vi "Frontend v3.0.vi"() -> ()   [LabVIEW 2016]
uses:
  Driver/Old driver/4155C Filename.vi
panel:
  in  "Panel Controls 2":T1={"Emergency Stop"=refnum, "CapGraph Max"=1e-05, "Text/Graph (text=false)"=FALSE} {"CapGraph Max" format="%.2e"}
  in  "Gate 3":T2={"Gate Start"=0.0, "Gate Stop"=2.0, "Gate Step"=1.0, "Gate Compliance"=0.0001, "Range mode"=0, "Range"=6} {"Range" max=11 scale=0.0..11.0; "Range mode" items=["Auto", "Limited", "Fixed"]; "Gate Compliance" min=0.0 max=0.1 format="%^.2e"; "Gate Step" min=-100.0 max=100.0 format="%^.4e"; "Gate Stop" min=-100.0 max=100.0 format="%^.4e"; "Gate Start" min=-100.0 max=100.0 format="%^.4e"}
  in  "Drain 3":T3={"Drain voltage"=0.0, "Drain Compliance"=0.0001, "Range mode"=0, "Range"=6} {"Range" max=11 scale=0.0..11.0; "Range mode" items=["Auto", "Limited", "Fixed"]; "Drain Compliance" min=0.0 max=0.1 format="%^.2e"; "Drain voltage" min=-100.0 max=100.0 format="%^.4e"}
  in  "Timings 2":T4={"hold time (sec)"=0.0, "delay time (sec)"=0.0, "Step Time (0 disables)"=0.0, "C-Step"=0.1, "CInt"=0.1, "IInt"=0.1} {"IInt" min=0.01 max=10.0 format="%.2f"; "CInt" min=0.01 max=10.0 format="%.2f"; "C-Step" min=0.01 max=10.0 format="%.2f"; "Step Time (0 disables)" min=0.0 format="%.2f"; "delay time (sec)" min=0.0 format="%.4f"; "hold time (sec)" min=0.0 format="%.4f"}
  in  "Gate 2":T5={"Gate Start"=0.0, "Gate Stop"=2.0, "Gate Step (linear only)"=1.0, "Gate Compliance"=0.0001, "Gate PComp"=0.0, "Range mode"=0, "Range"=6} {"Range" max=11 scale=0.0..11.0; "Range mode" items=["Auto", "Limited", "Fixed"]; "Gate PComp" format="%^.2e"; "Gate Compliance" format="%^.2e"; "Gate Step (linear only)" format="%^.4e"; "Gate Stop" format="%^.4e"; "Gate Start" format="%^.4e"}
  in  "Drain":T6={"Drain Start"=0.0, "Drain Stop"=2.0, "Drain Compliance"=0.0001, "Drain Step"=1.0, "Drain PComp"=0.0, "Range mode"=0, "Range"=6} {"Range" max=11 scale=0.0..11.0; "Range mode" items=["Auto", "Limited", "Fixed"]; "Drain PComp" format="%^.2e"; "Drain Step" format="%^.4e"; "Drain Compliance" format="%^.2e"; "Drain Stop" format="%^.4e"; "Drain Start" format="%^.4e"}
  in  "Gate":T7={"Gate Start"=0.0, "Gate Stop"=2.0, "Gate Step"=1.0, "Gate Compliance"=0.0001, "Gate PComp"=0.0, "Range mode"=0, "Range"=6} {"Range" max=11 scale=0.0..11.0; "Range mode" items=["Auto", "Limited", "Fixed"]; "Gate PComp" format="%^.2e"; "Gate Compliance" format="%^.2e"; "Gate Step" format="%^.4e"; "Gate Stop" format="%^.4e"; "Gate Start" format="%^.4e"}
  in  "Drain 2":T8={"Drain Start"=0.0, "Drain Stop"=2.0, "Drain Compliance"=0.0001, "Drain Step (linear only)"=1.0, "Drain PComp"=0.0, "Range mode"=0, "Range"=6} {"Range" max=11 scale=0.0..11.0; "Range mode" items=["Auto", "Limited", "Fixed"]; "Drain PComp" format="%^.2e"; "Drain Step (linear only)" format="%^.4e"; "Drain Compliance" format="%^.2e"; "Drain Stop" format="%^.4e"; "Drain Start" format="%^.4e"}
  in  "Timings":T9={"integration time"=0, "Short/Long integration time"=0.00064, "hold time (sec)"=0.0, "delay time (sec)"=0.0, "Step Time (0 disables)"=0.0, "sweep method"=0, "Pulse period"=0.005, "Base voltage"=0.0, "Pulse width"=0.0005} {"Pulse width" min=0.0005 max=0.1 step=0.0001 format="%.4f"; "Base voltage" format="%^.4e"; "Pulse period" min=0.005 max=1.0 step=0.0001 format="%.4f"; "sweep method" items=["Continuous", "Pulsed"]; "Step Time (0 disables)" format="%.2f"; "delay time (sec)" format="%.4f"; "hold time (sec)" format="%.4f"; "Short/Long integration time" format="%^.0e"; "integration time" scale=0.0..2.0}
  in  "Panel controls":T10={"Emergency Stop"=refnum, "OutputGraph Max"=1e-05, "Text/Graph (text=false)"=FALSE} {"OutputGraph Max" format="%.2e"}
  in  "Panel Controls":T11={"Emergency Stop"=refnum, "TransGraph Max"=1e-05, "Text/Graph (text=false)"=FALSE, "TransGraph Min"=1e-05} {"TransGraph Min" format="%.2e"; "TransGraph Max" format="%.2e"}
  in  "Tab Control":enum32{"Characteristics", "Other parameters"}(tab)
  in  "Drain Voltage":dbl min=-100.0 max=100.0 format="%.2f"
  in  "Cap voltage":dbl=0.1 min=0.0 max=10.0 format="%.2f"
  in  "Leak I-time":dbl=0.1 min=0.02 max=2.0 step=0.02 format="%.2f"
  in  "Cap I-time":dbl=0.1 min=0.04 max=400.0 step=0.02 format="%.2f"
  in  "QSCV Start":bool
  in  "Gate: Step 2":dbl=-2.0 format="%.2f"
  in  "Gate: Stop 2":dbl=-60.0 min=-100.0 max=100.0 format="%.2f"
  in  "Gate: Start 2":dbl min=-100.0 max=100.0 format="%.2f"
  in  "sweep method":u16(ring) items=["Continuous", "Pulsed"]
  out "Is":dbl format="%.2e"
  out "Id":dbl format="%.2e"
  out "Ig":dbl format="%.2e"
  in  "Vd":dbl(slide) min=-100.0 max=100.0 step=0.1 scale=-100.0..100.0 scale format="%.1f"
  in  "Vg":dbl(slide) min=-100.0 max=100.0 step=0.1 scale=-100.0..100.0 scale format="%.1f"
  in  "Real time sweep":bool
  in  "Interrupt run":bool
  in  "Running":bool=TRUE
  out "Path":path
  in  "integration time":u32(slide)=1 max=2 step=1 scale=0.0..2.0
  in  "sweep mode":u16(ring)=1 items=["Single", "Double"]
  in  "Transfer Start":bool
  in  "Output Start":bool
  in  "Drain: Step":dbl=1.0 min=-100.0 max=100.0 format="%.2f"
  in  "Drain: Stop":dbl=60.0 min=-100.0 max=100.0 format="%.2f"
  in  "Drain:Start":dbl min=-100.0 max=100.0 format="%.2f"
  in  "Gate: Step":dbl=10.0 min=-100.0 max=100.0 format="%.2f"
  in  "Gate: Stop":dbl=60.0 min=-100.0 max=100.0 format="%.2f"
  in  "Gate: Start":dbl min=-100.0 max=100.0 format="%.2f"
  out "XY Graph":cluster{"Y data in":dbl[], "X data in":dbl[]}[](graph)
  in  "Drain: Step":dbl=-55.0 min=-100.0 max=100.0 format="%.3f"
  in  "Drain: Stop":dbl=-60.0 min=-100.0 max=100.0 format="%.3f"
  in  "Drain:Start":dbl=-5.0 min=-100.0 max=100.0 format="%.3f"
  in  "Gate: Step":dbl=-1.0 min=-100.0 max=100.0 format="%.2f"
  in  "Gate: Stop":dbl=-60.0 min=-100.0 max=100.0 format="%.2f"
  in  "Gate: Start":dbl=10.0 min=-100.0 max=100.0 format="%.2f"
  in  "Gate: Compliance":dbl=0.001 min=1e-12 max=0.1 format="%.8f"
  in  "Drain: Compliance":dbl=0.01 min=1e-12 max=0.1 format="%.8f"
  in  "Drain":u32(ring)=1 items=["SMU1  ", "SMU2  ", "SMU3  ", "SMU4  ", "SMU5  ", "SMU6  ", "VSU1  ", "VSU2  "]
  in  "Source/Common":u32(ring) items=["SMU1  ", "SMU2  ", "SMU3  ", "SMU4  ", "SMU5  ", "SMU6  ", "VSU1  ", "VSU2  "]
  in  "Gate":u32(ring)=2 items=["SMU1  ", "SMU2  ", "SMU3  ", "SMU4  ", "SMU5  ", "SMU6  ", "VSU1  ", "VSU2  "]
  in  "Probe 4":u32(ring)=3 items=["SMU1  ", "SMU2  ", "SMU3  ", "SMU4  ", "SMU5  ", "SMU6  ", "VSU1  ", "VSU2  "]
  in  "TransGraph Min":dbl=1e-11 format="%.2e"
  in  "Logfile?":bool
  in  "Probe 4":cluster{"on/off":bool, "Voltage":dbl} {"Voltage" min=-100.0 max=100.0 format="%.2f"}
  in  "Pulse width":dbl=0.02 min=0.0005 max=0.1 step=0.0001 format="%.4f"
  in  "Base voltage":dbl min=-100.0 max=100.0 format="%.2f"
  in  "Pulse period":dbl=0.5 min=0.005 max=1.0 step=0.0001 format="%.4f"
  in  "Source/Drain\nRange":u8(slide)=3 max=11 scale=0.0..11.0
  in  "Source/Drain\nRange mode":u16(ring)=1 items=["Auto", "Limited", "Fixed"]
  in  "Gate Range":u8(slide)=3 max=11 scale=0.0..11.0
  in  "Gate Range\nmode":u16(ring)=1 items=["Auto", "Limited", "Fixed"]
  in  "Drain Power Compliance":dbl min=0.0 max=1.0 format="%.2f"
  in  "Gate Power\nCompliance":dbl min=0.0 max=1.0 format="%.2f"
  in  "OutputGraph Max":dbl=0.0001 format="%.2e"
  in  "TransGraph Max":dbl=0.001 format="%.2e"
  in  "SPA Display":bool=TRUE
  in  "Step delay /s":dbl min=0.0 max=1.0 format="%.2f"
  in  "Integration time (long)":dbl=0.32 min=0.04 max=2.0 step=0.02 format="%.2f"
  in  "Integration time (short)":dbl=0.00096 min=8e-05 max=0.00192 step=8e-05 format="%^.0e"
  in  "hold time /s":dbl min=0.0 max=655.35 step=0.01 format="%.2f"
  in  "delay time /s":dbl min=0.0 max=65.535 step=0.0001 format="%.2f"
  in  "Decimal places in header":i8=1
  out "error out":errorcluster
  in  "VISA resource name in":refnum<visa-resource-name>="GPIB0::14::INSTR"
  in  "Standby":T12
  # "Transfer Characteristics"
  # "V"
  # "V"
  # "V"
  # "Gate"
  # "V"
  # "V"
  # "Drain"
  # "V"
  # "Output Characteristics"
  # "V"
  # "V"
  # "V"
  # "Gate"
  # "V"
  # "V"
  # "Drain"
  # "V"
  # "Quasi Static Capacitance measurement"
  # "V"
  # "V"
  # "V"
  # "Gate"
  # "s"
  # "V"
  # "V"
  # "s"
  # "A"
  # "A"
  # "Pulsed mode settings"
  # "s"
  # "NOTE - THIS OVERRIDES THE COMPLIANCE VALUES!"
  # "s"
  # "A"
  # "Enter max power in Watts (max 1W)"
  # "A"
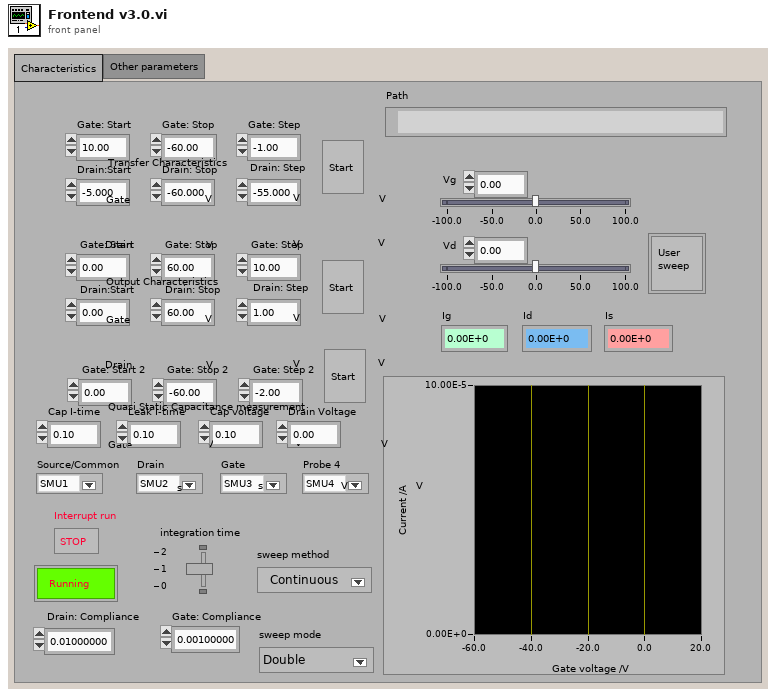
[diagram p1: front panel]
types:
  T1 = cluster{"Emergency Stop":refnum<vi>, "CapGraph Max":dbl, "Text/Graph (text=false)":bool}
  T2 = cluster{"Gate Start":dbl, "Gate Stop":dbl, "Gate Step":dbl, "Gate Compliance":dbl, "Range mode":u16, "Range":u8}
  T3 = cluster{"Drain voltage":dbl, "Drain Compliance":dbl, "Range mode":u16, "Range":u8}
  T4 = cluster{"hold time (sec)":dbl, "delay time (sec)":dbl, "Step Time (0 disables)":dbl, "C-Step":dbl, "CInt":dbl, "IInt":dbl}
  T5 = cluster{"Gate Start":dbl, "Gate Stop":dbl, "Gate Step (linear only)":dbl, "Gate Compliance":dbl, "Gate PComp":dbl, "Range mode":u16, "Range":u8}
  T6 = cluster{"Drain Start":dbl, "Drain Stop":dbl, "Drain Compliance":dbl, "Drain Step":dbl, "Drain PComp":dbl, "Range mode":u16, "Range":u8}
  T7 = cluster{"Gate Start":dbl, "Gate Stop":dbl, "Gate Step":dbl, "Gate Compliance":dbl, "Gate PComp":dbl, "Range mode":u16, "Range":u8}
  T8 = cluster{"Drain Start":dbl, "Drain Stop":dbl, "Drain Compliance":dbl, "Drain Step (linear only)":dbl, "Drain PComp":dbl, "Range mode":u16, "Range":u8}
  T9 = cluster{"integration time":u32, "Short/Long integration time":dbl, "hold time (sec)":dbl, "delay time (sec)":dbl, "Step Time (0 disables)":dbl, "sweep method":u16, "Pulse period":dbl, "Base voltage":dbl, "Pulse width":dbl}
  T10 = cluster{"Emergency Stop":refnum<vi>, "OutputGraph Max":dbl, "Text/Graph (text=false)":bool}
  T11 = cluster{"Emergency Stop":refnum<vi>, "TransGraph Max":dbl, "Text/Graph (text=false)":bool, "TransGraph Min":dbl}
  T12 = cluster{"Gate Standby":bool, "Drain Standby":bool}
  T13 = cluster{"V2 Start":dbl, "V2 Step":dbl, "Number of points":i32}
  T14 = enum16{"open", "replace", "create", "open or create", "replace or create", "replace or create with confirmation"}
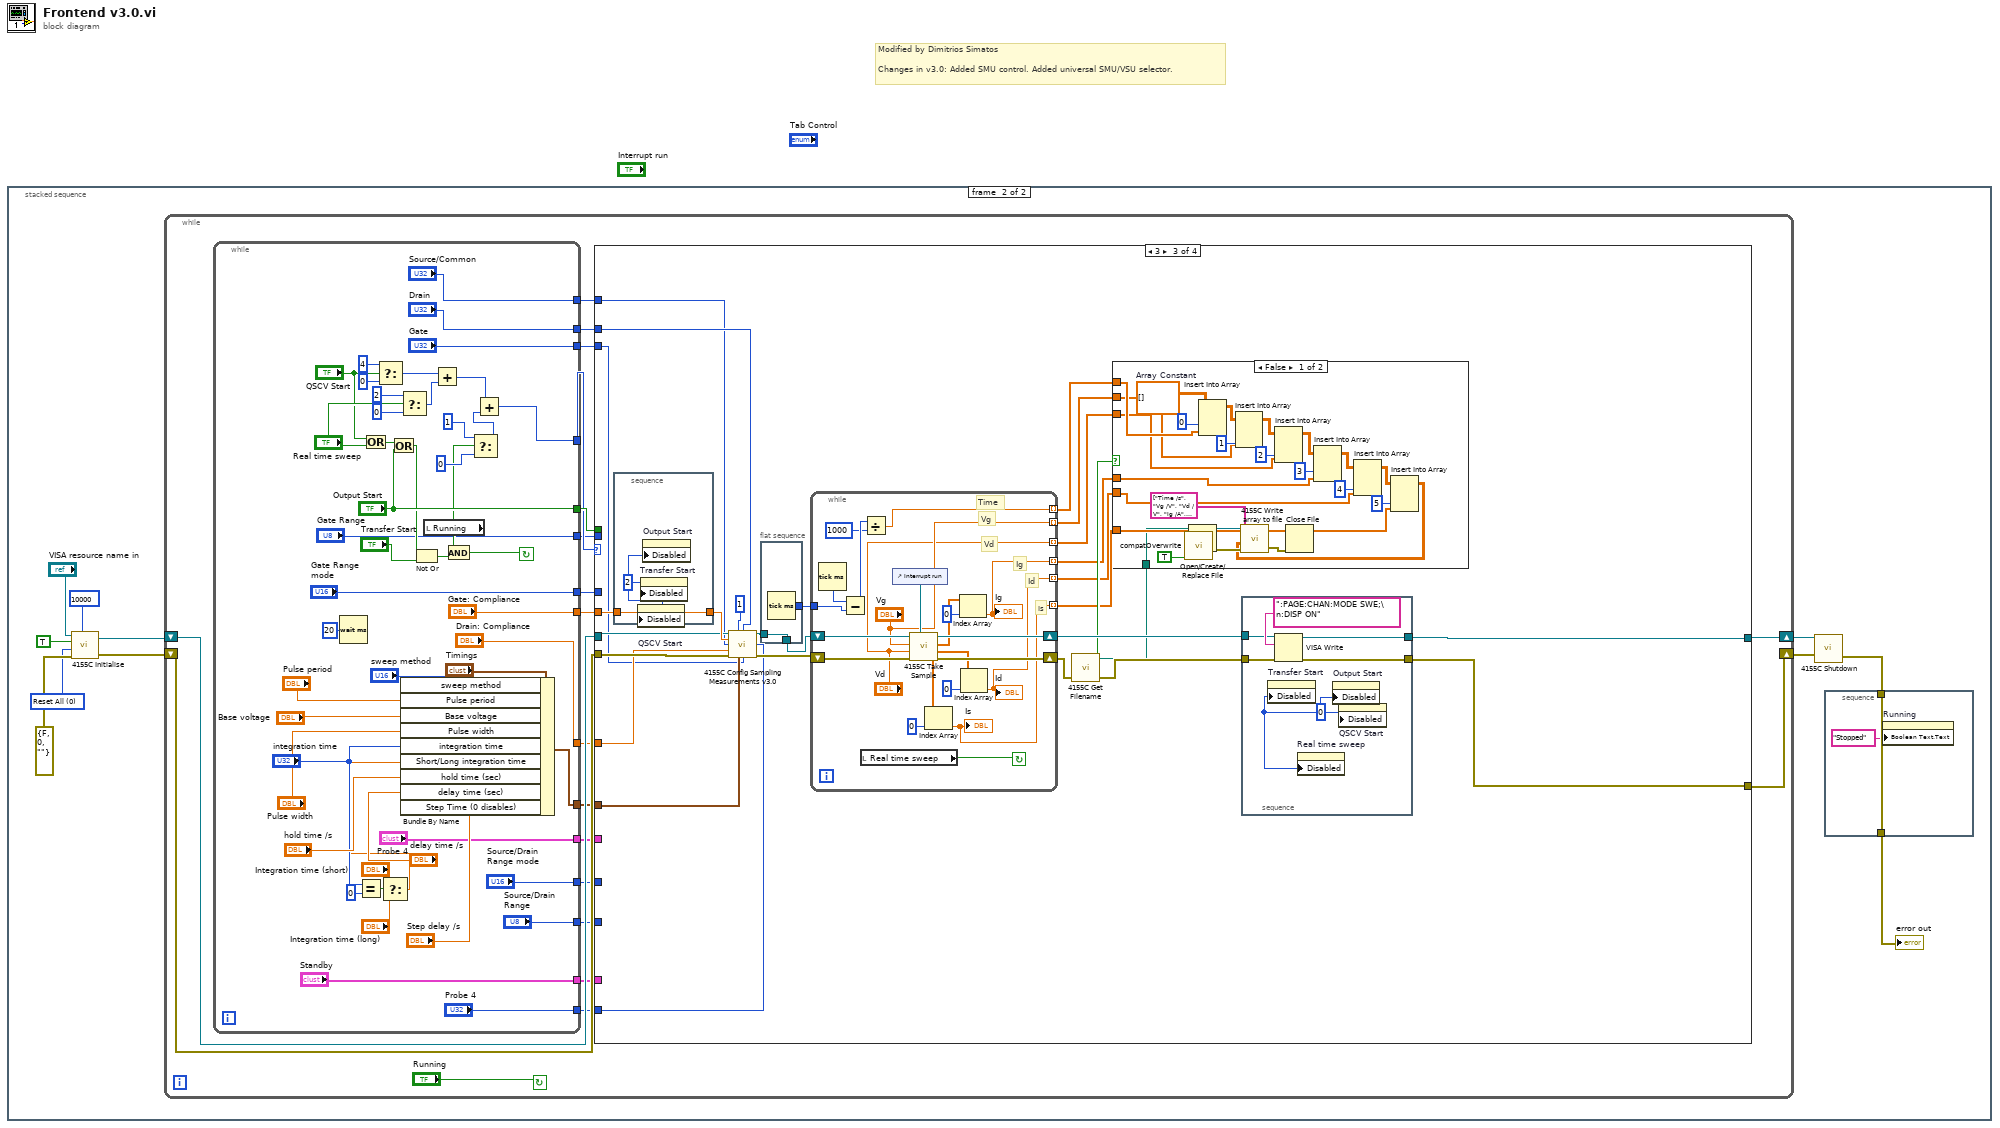
[diagram p0: block diagram]
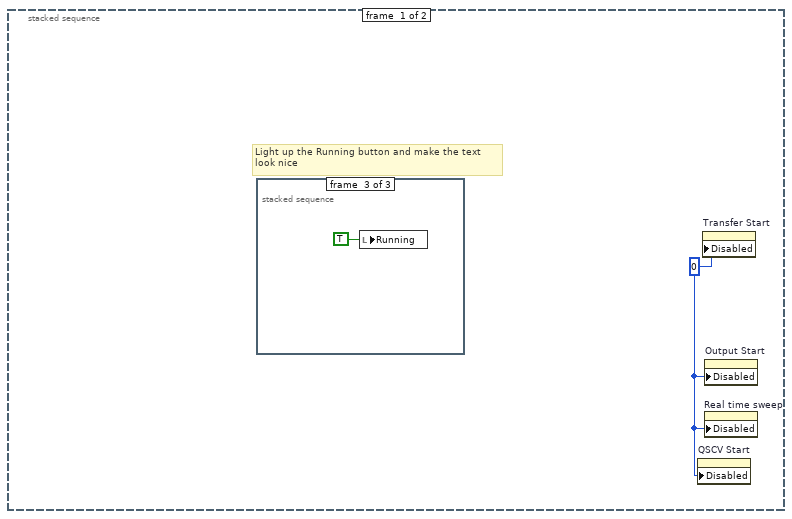
[diagram p2: hidden frame]
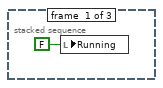
[diagram p3: hidden frame]
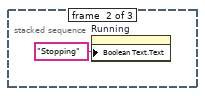
[diagram p4: hidden frame]
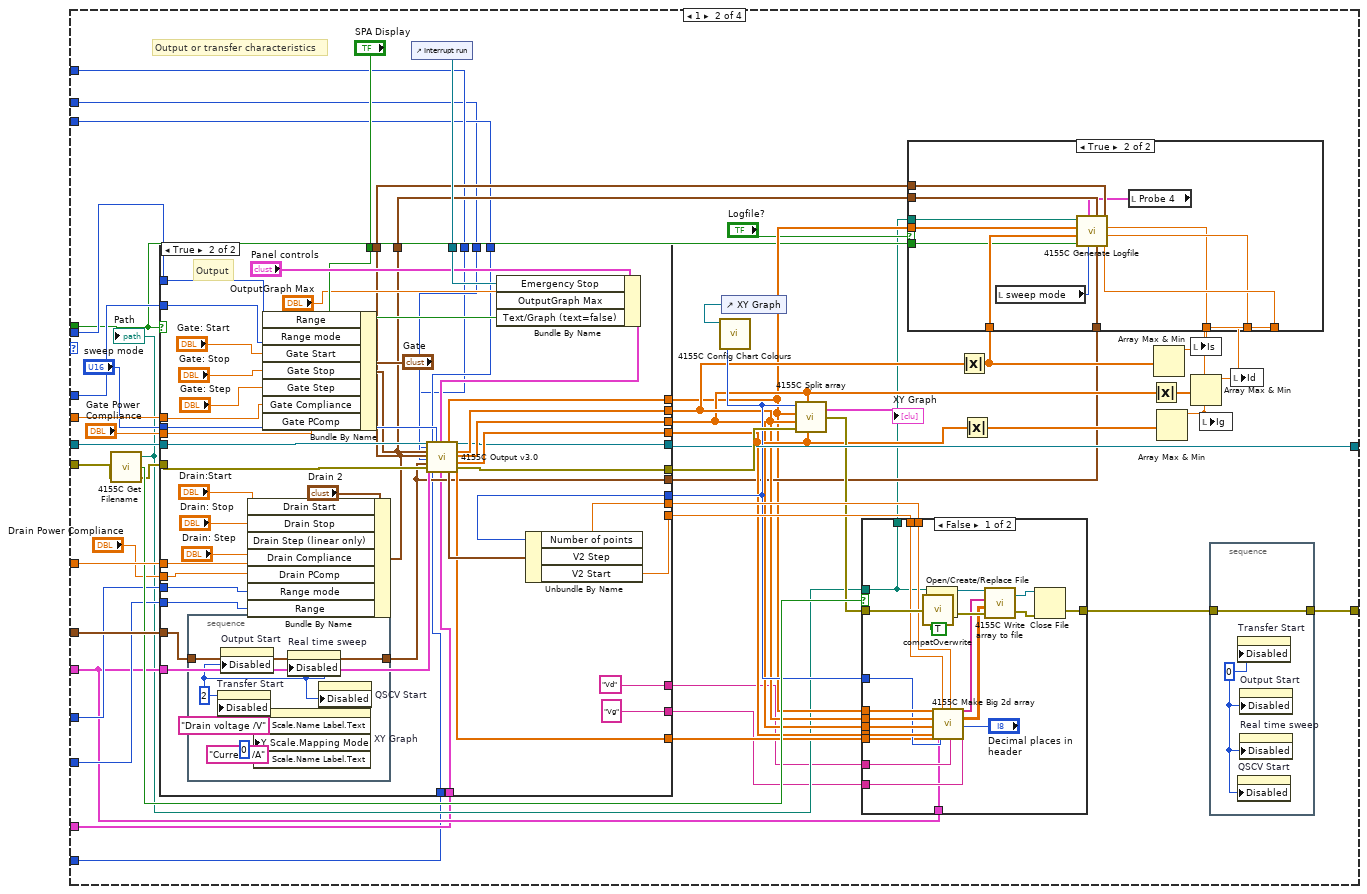
[diagram p6: hidden frame]
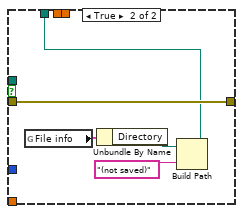
[diagram p8: hidden frame]
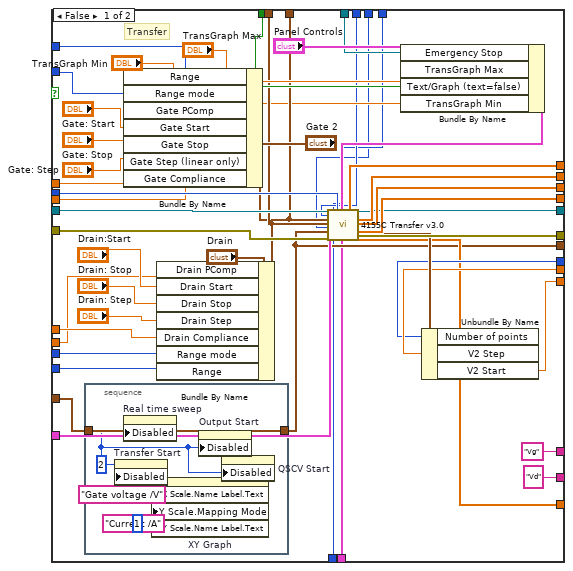
[diagram p9: hidden frame]
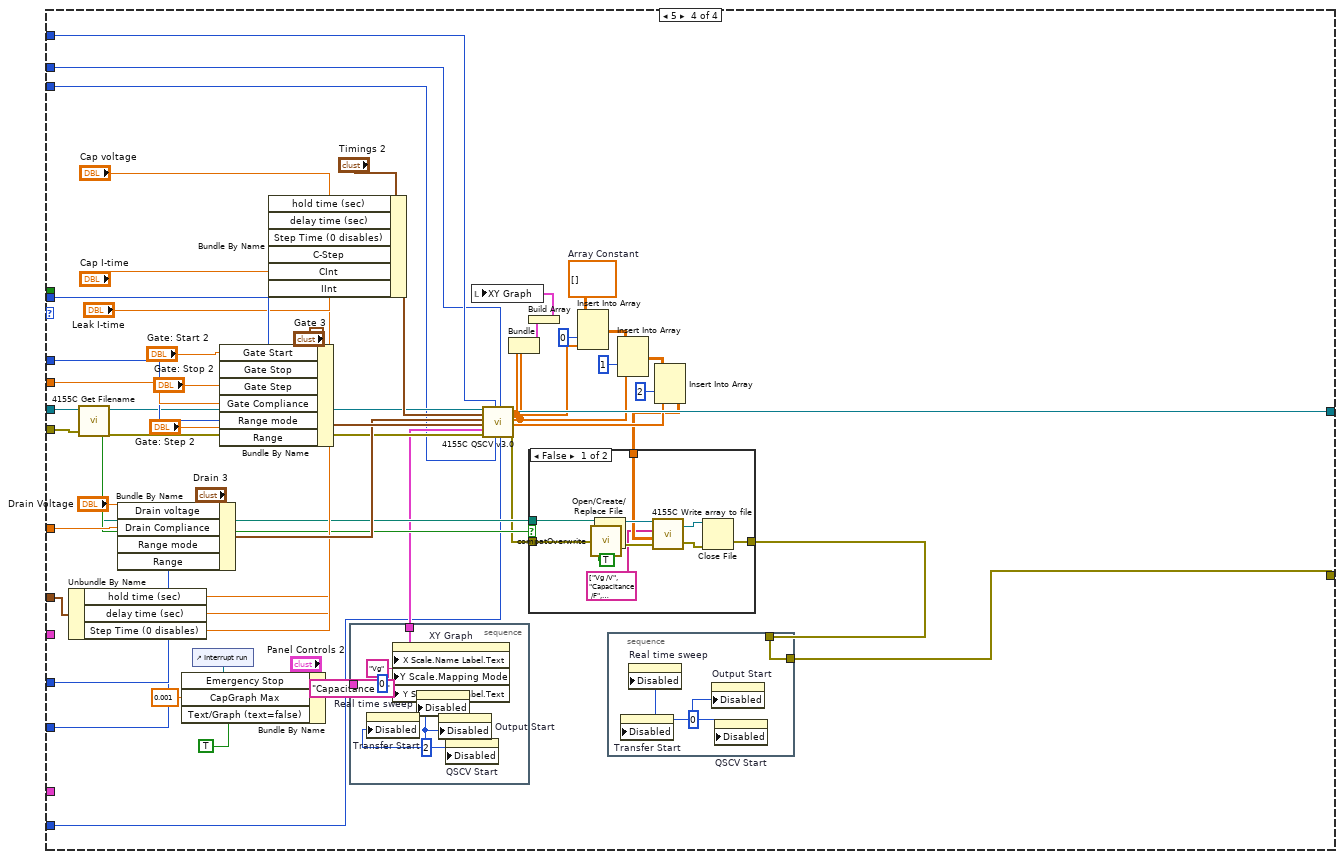
[diagram p11: hidden frame]
diagram:
  # "Modified by Dimitrios Simatos\n\nChanges in v3.0: Added SMU control. Added universal SMU/VSU selector."
  n1 = stacked-sequence {
    frame #0 {
      w1 = u8 0 ("Disabled")
      # "Light up the Running button and make the text\nlook nice"
      n2 = stacked-sequence {
        frame #0 {
          n3 = local write "Running"(FALSE ("Running")) -> ()
        }
        frame #1 {
          n4 = property on="Running" class="Bool (strict)"("Boolean Text.Text"="Stopping") -> ()  [unwired: 2 in, 2 out]
        }
        frame #2 {
          (unwired) FALSE ("Running")
          n5 = local write "Running"(TRUE ("Running")) -> ()
        }
      }
      n6 = property on="QSCV Start" class="Bool (strict)"("Disabled"=w1) -> ()  [unwired: 2 in, 2 out]
      n7 = property on="Transfer Start" class="Bool (strict)"("Disabled"=w1) -> ()  [unwired: 2 in, 2 out]
      n8 = property on="Output Start" class="Bool (strict)"("Disabled"=w1) -> ()  [unwired: 2 in, 2 out]
      n9 = property on="Real time sweep" class="Bool (strict)"("Disabled"=w1) -> ()  [unwired: 2 in, 2 out]
    }
    frame #1 {
      w11 = u16 0 items=["Reset All", "Partial reset"] ("Type of reset")
      n10 = call "4155C Initialise.vi"("VISA resource name in"="VISA resource name in", "Reset"=TRUE, "Type of reset"=w11, "error in (no error)"=errorcluster {"status"=FALSE, "code"=0, "source"=""}, "VISA Timeout Value"=u32 10000) -> ("VISA Resource Name out"=w10:refnum<visa-resource-name>, "error out"=w9:errorcluster)
      n11 = while {
        shift-left: w10 -> [w30]
        shift-right: [w32] -> w5
        shift-left: w9 -> [w31]
        shift-right: [w33] -> w6
        stop <- "Running" continue-if-true
        n12 = while {
          tunnel: ["Probe 4"] -> w21
          tunnel: ["Gate Range"] -> w22
          tunnel: ["Gate Range\nmode"] -> w23
          tunnel: ["Source/Drain\nRange"] -> w24
          tunnel: ["Source/Drain\nRange mode"] -> w25
          tunnel: ["Drain: Compliance"] -> w26
          tunnel: [w41] -> w27
          tunnel: ["Gate: Compliance"] -> w28
          tunnel: [w73] -> w29
          tunnel: ["Output Start"] -> w34
          tunnel: ["Standby"] -> w20
          tunnel: ["Source/Common"] -> w19
          tunnel: ["Gate"] -> w18
          tunnel: ["Drain"] -> w17
          tunnel: ["Probe 4"] -> w16
          stop <- w82 continue-if-true
          n13 = Wait (ms)(milliseconds to wait=u32 20) -> ()  [unwired: 1 out]
          n14 = Equal?(x="integration time", y=u32 0) -> (x = y?=w65:bool)
          n15 = Or(x="QSCV Start", y="Real time sweep") -> (x .or. y?=w53:bool)
          n16 = Select(t=i8 4, s="QSCV Start", f=i8 0) -> (s? t:f=w48:i8)
          n17 = Select(t="Integration time (short)", s=w65, f="Integration time (long)") -> (s? t:f=w62:dbl)
          n18 = Or(x=w53, y="Output Start") -> (x .or. y?=w79:bool)
          n19 = Select(t=i8 2, s="Real time sweep", f=i8 0) -> (s? t:f=w49:i8)
          n20 = Bundle By Name(cluster="Timings", "sweep method"="sweep method", "Pulse period"="Pulse period", "Base voltage"="Base voltage", "Pulse width"="Pulse width", "integration time"="integration time", "Short/Long integration time"=w62, "hold time (sec)"="hold time /s", "delay time (sec)"="delay time /s", "Step Time (0 disables)"="Step delay /s") -> (w41:T9)
          n21 = Not Or(1:"Transfer Start", 2:w79) -> (0:w81:bool)
          n22 = local read "Running"() -> (w76:bool)
          n23 = Add(x=w48, y=w49) -> (x+y=w47:i8)
          n24 = And(x=w76, y=w81) -> (x .and. y?=w82:bool)
          n25 = Select(t=i8 1, s=w76, f=i8 0) -> (s? t:f=w72:i8)
          n26 = Add(x=w47, y=w72) -> (x+y=w73:i8)
        }
        n27 = case shown="3" w29 {
          tunnel: w34 -> [_ w96 _ _]
          tunnel: w27 -> [_ w137 w302 w405]
          tunnel: w28 -> [_ w136 w312 w417]
          tunnel: w26 -> [_ w135 w306 w421]
          tunnel: [w85 w128 w310 w376] -> w33
          tunnel: [w84 w131 w311 w401] -> w32
          tunnel: w31 -> [w85 w122 w308 w397]
          tunnel: w30 -> [w84 w130 w307 w396]
          tunnel: w25 -> [_ w107 _ w414]
          tunnel: w24 -> [_ w106 _ w413]
          tunnel: w23 -> [_ w105 _ w416]
          tunnel: w22 -> [_ w104 _ w415]
          tunnel: w21 -> [_ w102 _ _]
          tunnel: w20 -> [_ w90 _ _]
          tunnel: w19 -> [_ w89 w287 w373]
          tunnel: w18 -> [_ w88 w286 w374]
          tunnel: w17 -> [_ w87 w288 w372]
          tunnel: w16 -> [_ w86 w285 w375]
          frame 0, Default {
            # "Someone's deselected the running button so just shutdown..."
          }
          frame 1 {
            # "Output or transfer characteristics"
            n28 = call "4155C Get Filename.vi"("error in (no error)"=w122) -> ("error out"=w121:errorcluster, "cancelled"=w127:bool, "path"=w95:path)  [unwired: 2 in]
            "Path" <- w95
            n29 = control-ref of="Interrupt run"() -> (w123:refnum<vi>)
            n30 = case shown="True" w96 {
              tunnel: w130 -> [w209 w261]
              tunnel: w121 -> [w208 w260]
              tunnel: w137 -> [w212 w266]
              tunnel: w136 -> [w222 w277]
              tunnel: w135 -> [w227 w276]
              tunnel: "sweep mode" -> [w221 w275]
              tunnel: [w220 w274] -> w97
              tunnel: [w219 w273] -> w109
              tunnel: [w218 w272] -> w108
              tunnel: [w217 w271] -> w110
              tunnel: [w216 w270] -> w131
              tunnel: [w215 w269] -> w134
              tunnel: [w192 w245] -> w126
              tunnel: [w193 w244] -> w132
              tunnel: [w185 w243] -> w133
              tunnel: ["Vg" "Vd"] -> w92
              tunnel: ["Vd" "Vg"] -> w91
              tunnel: w123 -> [w206 w259]
              tunnel: "SPA Display" -> [w205 w257]
              tunnel: "Drain Power Compliance" -> [w201 w254]
              tunnel: "Gate Power\nCompliance" -> [w202 w253]
              tunnel: w107 -> [w196 w250]
              tunnel: w106 -> [w195 w249]
              tunnel: w105 -> [w197 w248]
              tunnel: w104 -> [w198 w247]
              tunnel: w102 -> [w191 w242]
              tunnel: [w190 w241] -> w103
              tunnel: [w189 w239] -> w100
              tunnel: [w188 w240] -> w99
              tunnel: [w187 w238] -> w98
              tunnel: w90 -> [w184 w233]
              tunnel: w89 -> [w183 w235]
              tunnel: w88 -> [w182 w237]
              tunnel: w87 -> [w181 w236]
              tunnel: w86 -> [w180 w234]
              frame False {
                # "Transfer"
                n31 = stacked-sequence {
                  tunnel: w212 -> [w231]
                  tunnel: [w231] -> w187
                  frame #0 {
                    w229 = u8 2 ("Disabled")
                    n32 = property on="Transfer Start" class="Bool (strict)"("Disabled"=w229) -> ()  [unwired: 2 in, 2 out]
                    n33 = property on="Real time sweep" class="Bool (strict)"("Disabled"=w229) -> ()  [unwired: 2 in, 2 out]
                    n34 = property on="XY Graph" class="XYGraph (strict)"("X Scale.Name Label.Text"="Gate voltage /V", "Y Scale.Mapping Mode"=u8 1, "Y Scale.Name Label.Text"="Current /A") -> ()  [unwired: 2 in, 2 out]
                    n35 = property on="Output Start" class="Bool (strict)"("Disabled"=w229) -> ()  [unwired: 2 in, 2 out]
                    n36 = property on="QSCV Start" class="Bool (strict)"("Disabled"=w229) -> ()  [unwired: 2 in, 2 out]
                  }
                }
                n37 = Bundle By Name(cluster="Gate 2", "Range"=w198, "Range mode"=w197, "Gate PComp"=w202, "Gate Start"="Gate: Start", "Gate Stop"="Gate: Stop", "Gate Step (linear only)"="Gate: Step", "Gate Compliance"=w222) -> (w188:T5)
                n38 = Bundle By Name(cluster="Drain", "Drain PComp"=w201, "Drain Start"="Drain:Start", "Drain Stop"="Drain: Stop", "Drain Step"="Drain: Step", "Drain Compliance"=w227, "Range mode"=w196, "Range"=w195) -> (w189:T6)
                n39 = Bundle By Name(cluster="Panel Controls", "Emergency Stop"=w206, "TransGraph Max"="TransGraph Max", "Text/Graph (text=false)"=w205, "TransGraph Min"="TransGraph Min") -> (w203:T11)
                n40 = call "4155C Transfer v3.0.vi"("VISA resource name in"=w209, "Source/Common"=w183, 2:"Gate"=w188, 3:"Drain"=w189, 4:"Drain"=w181, "Timings"=w187, "error in (no error)"=w208, 7:"Probe 4"=w191, 8:"Gate"=w182, 9:"Probe 4"=w180, "sweep mode"=w221, "Panel Controls"=w203, "Standby"=w184) -> ("VG"=w220:dbl[], "Outparams"=w194:T13, "VISA Resource Name out"=w216:refnum<visa-resource-name>, "IS"=w219:dbl[], "ID"=w218:dbl[], "IG"=w217:dbl[], "error out"=w215:errorcluster, "Probe 4"=w190:dbl[])  [unwired: 7 in]
                n41 = Unbundle By Name(w194) -> ("Number of points"=w192:i32, "V2 Step"=w193:dbl, "V2 Start"=w185:dbl)
              }
              frame True {
                # "Output"
                n42 = stacked-sequence {
                  tunnel: w266 -> [w283]
                  tunnel: [w283] -> w238
                  frame #0 {
                    w281 = u8 2 ("Disabled")
                    n43 = property on="Transfer Start" class="Bool (strict)"("Disabled"=w281) -> ()  [unwired: 2 in, 2 out]
                    n44 = property on="Output Start" class="Bool (strict)"("Disabled"=w281) -> ()  [unwired: 2 in, 2 out]
                    n45 = property on="XY Graph" class="XYGraph (strict)"("X Scale.Name Label.Text"="Drain voltage /V", "Y Scale.Mapping Mode"=u8 0, "Y Scale.Name Label.Text"="Current /A") -> ()  [unwired: 2 in, 2 out]
                    n46 = property on="Real time sweep" class="Bool (strict)"("Disabled"=w281) -> ()  [unwired: 2 in, 2 out]
                    n47 = property on="QSCV Start" class="Bool (strict)"("Disabled"=w281) -> ()  [unwired: 2 in, 2 out]
                  }
                }
                n48 = Bundle By Name(cluster="Drain 2", "Drain Start"="Drain:Start", "Drain Stop"="Drain: Stop", "Drain Step (linear only)"="Drain: Step", "Drain Compliance"=w276, "Drain PComp"=w254, "Range mode"=w250, "Range"=w249) -> (w239:T8)
                n49 = Bundle By Name(cluster="Gate", "Range"=w247, "Range mode"=w248, "Gate Start"="Gate: Start", "Gate Stop"="Gate: Stop", "Gate Step"="Gate: Step", "Gate Compliance"=w277, "Gate PComp"=w253) -> (w240:T7)
                n50 = Bundle By Name(cluster="Panel controls", "Emergency Stop"=w259, "OutputGraph Max"="OutputGraph Max", "Text/Graph (text=false)"=w257) -> (w255:T10)
                n51 = call "4155C Output v3.0.vi"("VISA resource name in"=w261, "Source/Common"=w235, 2:"Gate"=w240, 3:"Drain"=w239, 4:"Drain"=w236, "Timings"=w238, "error in (no error)"=w260, 7:"Probe 4"=w242, 8:"Gate"=w237, 9:"Probe 4"=w234, "sweep mode"=w275, "Panel controls"=w255, "Standby"=w233) -> ("VD"=w274:dbl[], "Outparams"=w246:T13, "VISA Resource Name out"=w270:refnum<visa-resource-name>, "IS"=w273:dbl[], "ID"=w272:dbl[], "IG"=w271:dbl[], "error out"=w269:errorcluster, "Probe 4"=w241:dbl[])  [unwired: 7 in]
                n52 = Unbundle By Name(w246) -> ("Number of points"=w245:i32, "V2 Step"=w244:dbl, "V2 Start"=w243:dbl)
              }
            }
            n53 = control-ref of="XY Graph"() -> (w124:refnum<vi>)
            n54 = call "4155C Config Chart Colours.vi"("Numeric"=w126, "XY Graph 2"=w124) -> ()  [unwired: 6 in]
            n55 = call "4155C Split array.vi"("Number of VAR2 steps"=w126, "Y2 data in"=w108, "X data in"=w97, "Y1 data in"=w109, "Y3 data in"=w110, "error in (no error)"=w134) -> ("Array of clusters"=→"XY Graph":cluster{"Y data in":dbl[], "X data in":dbl[]}[], "error out"=w120:errorcluster)  [unwired: 1 in]
            n56 = case shown="False" w127 {
              tunnel: w120 -> [w173 w179]
              tunnel: [w169 w179] -> w129
              tunnel: w95 -> [w153 _]
              tunnel: w126 -> [w163 _]
              tunnel: w108 -> [w165 _]
              tunnel: w97 -> [w167 _]
              tunnel: w109 -> [w166 _]
              tunnel: w110 -> [w164 _]
              tunnel: w133 -> [w157 _]
              tunnel: w132 -> [w158 _]
              tunnel: w92 -> [w162 _]
              tunnel: w91 -> [w161 _]
              tunnel: w103 -> [w155 _]
              tunnel: w102 -> [w154 _]
              tunnel: [w153 w175] -> w93
              frame False {
                n57 = call <vilib>:"compatOverwrite.vi"("overwrite (F)"=TRUE) -> ("overwrite?"=w152:T14)
                n58 = Open/Create/Replace File(file path (use dialog)=w153, error in=w173, operation (0:open)=w152) -> (refnum out=w171:refnum<file>, error out=w172:errorcluster)  [unwired: 3 in, 1 out]
                n59 = call "4155C Make Big 2d array.vi"("1D Var1"=w167, "1d IS"=w166, "1d ID"=w165, "1d IG"=w164, "1d SMU4"=w155, "SMU4"=w154, "VAR2 START"=w157, "Number of VAR2 steps"=w163, "VAR2 STEP"=w158, "VAR1 Name"=w162, "Decimal places in header"="Decimal places in header", "VAR2 Name"=w161) -> ("Header array"=w159:string[], "Data array"=w160:dbl[][])  [unwired: 14 in]
                n60 = call "4155C Write array to file.vi"("Byte Stream File Refnum"=w171, "Header"=w159, "Data Array"=w160, "error in (no error)"=w172) -> ("dup refnum"=w168:refnum<file>, "error out"=w170:errorcluster)  [unwired: 1 in]
                n61 = Close File(refnum=w168, error in=w170) -> (error out=w169:errorcluster)  [unwired: 1 out]
              }
              frame True {
                n62 = global read "4155C Filename.vi" "File info"() -> (w178:cluster{"Filename":string, "Directory":path})
                n63 = Unbundle By Name(w178) -> ("Directory"=w177:path)
                n64 = Build Path(base path=w177, name or relative path="(not saved)") -> (appended path=w175:path)
              }
            }
            n65 = Absolute Value(x=w109) -> (abs(x)=w101:dbl[])
            n66 = Absolute Value(x=w110) -> (abs(x)=w115:dbl[])
            n67 = Absolute Value(x=w108) -> (abs(x)=w114:dbl[])
            n68 = Array Max & Min(array=w101) -> (max value=w112:dbl)  [unwired: 3 out]
            n69 = Array Max & Min(array=w115) -> (max value=w113:dbl)  [unwired: 3 out]
            n70 = local write "Is"(w112) -> ()
            n71 = Array Max & Min(array=w114) -> (max value=w111:dbl)  [unwired: 3 out]
            n72 = case shown="True" "Logfile?" {
              tunnel: w101 -> [_ w146]
              tunnel: w112 -> [_ w142]
              tunnel: w111 -> [_ w143]
              tunnel: w113 -> [_ w144]
              tunnel: w100 -> [_ w149]
              tunnel: w99 -> [_ w148]
              tunnel: w98 -> [_ w147]
              tunnel: w97 -> [_ w145]
              tunnel: w93 -> [_ w139]
              tunnel: w96 -> [_ w138]
              frame False {
              }
              frame True {
                n73 = local read "sweep mode"() -> (w140:u16)
                n74 = local read "Probe 4"() -> (w141:cluster{"on/off":bool, "Voltage":dbl})
                n75 = call "4155C Generate Logfile.vi"("Ig"=w144, "Id"=w143, "Is"=w142, "Drain"=w149, "Timings"=w147, "Gate"=w148, "sweep mode"=w140, "SMU4"=w141, "Output?"=w138, "Input I"=w146, "VG"=w145, "Path"=w139) -> ()
              }
            }
            n76 = local write "Ig"(w113) -> ()
            n77 = stacked-sequence {
              tunnel: w129 -> [w151]
              tunnel: [w151] -> w128
              frame #0 {
                w150 = u8 0 ("Disabled")
                n78 = property on="Transfer Start" class="Bool (strict)"("Disabled"=w150) -> ()  [unwired: 2 in, 2 out]
                n79 = property on="QSCV Start" class="Bool (strict)"("Disabled"=w150) -> ()  [unwired: 2 in, 2 out]
                n80 = property on="Output Start" class="Bool (strict)"("Disabled"=w150) -> ()  [unwired: 2 in, 2 out]
                n81 = property on="Real time sweep" class="Bool (strict)"("Disabled"=w150) -> ()  [unwired: 2 in, 2 out]
              }
            }
            n82 = local write "Id"(w111) -> ()
          }
          frame 3 {
            n83 = stacked-sequence {
              tunnel: w312 -> [w371]
              tunnel: [w371] -> w309
              frame #0 {
                w370 = u8 2 ("Disabled")
                n84 = property on="QSCV Start" class="Bool (strict)"("Disabled"=w370) -> ()  [unwired: 2 in, 2 out]
                n85 = property on="Transfer Start" class="Bool (strict)"("Disabled"=w370) -> ()  [unwired: 2 in, 2 out]
                n86 = property on="Output Start" class="Bool (strict)"("Disabled"=w370) -> ()  [unwired: 2 in, 2 out]
              }
            }
            n87 = call "4155C Config Sampling Measurements v3.0.vi"("VISA session"=w307, "Num Points"=i16 1, "Sample - Drain"=w288, "Gate Compliance"=w309, "Sample - Source/Common"=w287, "Sample - Probe 4"=w285, "Drain Compliance"=w306, "error in (no error)"=w308, "Timings"=w302, "Sample - Gate"=w286) -> ("dup VISA resource name"=w300:refnum<visa-resource-name>, "error out"=w304:errorcluster)  [unwired: 4 in]
            n88 = flat-sequence {
              tunnel: [w341] -> w301
              tunnel: w300 -> [w341]
              tunnel: [w340] -> w299
              frame #0 {
                n89 = Tick Count (ms)() -> (millisecond timer value=w340:u32)
              }
            }
            n90 = while {
              shift-left: w304 -> [w361]
              shift-right: [w360] -> w298
              shift-left: w301 -> [w362]
              shift-right: [w359] -> w305
              tunnel: ["Vg"] -> w293 mode=indexing
              tunnel: ["Vd"] -> w292 mode=indexing
              tunnel: [w349] -> w291 mode=indexing
              tunnel: [w348] -> w290 mode=indexing
              tunnel: [w347] -> w289 mode=indexing
              tunnel: w299 -> [w345]
              tunnel: [w342] -> w294 mode=indexing
              stop <- w363 continue-if-true
              # "Is"
              # "Id"
              # "Ig"
              # "Vd"
              # "Vg"
              # "Time"
              n91 = Tick Count (ms)() -> (millisecond timer value=w346:u32)
              n92 = Subtract(x=w346, y=w345) -> (x-y=w344:u32)
              n93 = local read "Real time sweep"() -> (w363:bool)
              n94 = Divide(x=w344, y=u32 1000) -> (x/y=w342:dbl)
              n95 = control-ref of="Interrupt run"() -> (w358:refnum<vi>)
              n96 = call "4155C Take Sample.vi"("Emergency Stop"=w358, "error in (no error)"=w361, "Vd"="Vd", "Vg"="Vg", "VISA resource name in"=w362) -> ("error out"=w360:errorcluster, "Id"=w354:dbl[], "Ig"=w352:dbl[], "VISA Resource Name out"=w359:refnum<visa-resource-name>, "Is"=w356:dbl[])  [unwired: 1 in, 1 out]
              n97 = Index Array(array=w356, index=0 ("Index")) -> (element=w347:dbl)
              "Is" <- w347
              n98 = Index Array(array=w352, index=0 ("Index")) -> (element=w349:dbl)
              "Ig" <- w349
              n99 = Index Array(array=w354, index=0 ("Index")) -> (element=w348:dbl)
              "Id" <- w348
            }
            n100 = call "4155C Get Filename.vi"("error in (no error)"=w298) -> ("error out"=w297:errorcluster, "cancelled"=w296:bool, "path"=w295:path)  [unwired: 2 in]
            n101 = case shown="False" w296 {
              tunnel: w295 -> [w320 _]
              tunnel: w294 -> [w337 _]
              tunnel: w293 -> [w328 _]
              tunnel: w292 -> [w327 _]
              tunnel: w291 -> [w326 _]
              tunnel: w290 -> [w325 _]
              tunnel: w289 -> [w322 _]
              frame False {
                w339 = dbl[][] []  # Array Constant
                n102 = call <vilib>:"compatOverwrite.vi"("overwrite (F)"=TRUE) -> ("overwrite?"=w313:T14)
                n103 = Open/Create/Replace File(file path (use dialog)=w320, operation (0:open)=w313) -> (refnum out=w318:refnum<file>, error out=w319:errorcluster)  [unwired: 4 in, 1 out]
                n104 = Insert Into Array(array=w339, index (col)=0 ("Disabled Index (col)"), new element=w337) -> (w336:dbl[][])  [unwired: 1 in]
                n105 = Insert Into Array(array=w336, index (col)=1 ("disabled index (col)"), new element=w328) -> (w335:dbl[][])  [unwired: 1 in]
                n106 = Insert Into Array(array=w335, index (col)=2 ("disabled index (col)"), new element=w327) -> (w334:dbl[][])  [unwired: 1 in]
                n107 = Insert Into Array(array=w334, index (col)=3 ("disabled index (col)"), new element=w326) -> (w333:dbl[][])  [unwired: 1 in]
                n108 = Insert Into Array(array=w333, index (col)=4 ("disabled index (col)"), new element=w325) -> (w324:dbl[][])  [unwired: 1 in]
                n109 = Insert Into Array(array=w324, index (col)=5 ("disabled index (col)"), new element=w322) -> (w316:dbl[][])  [unwired: 1 in]
                n110 = call "4155C Write array to file.vi"("Byte Stream File Refnum"=w318, "Header"=string[] ["Time /s", "Vg /V", "Vd /V", "Ig /A", "Id /A", "Is /A"], "Data Array"=w316, "error in (no error)"=w319) -> ("dup refnum"=w317:refnum<file>, "error out"=w321:errorcluster)  [unwired: 1 in]
                n111 = Close File(refnum=w317, error in=w321) -> ()  [unwired: 2 out]
              }
              frame True {
              }
            }
            n112 = stacked-sequence {
              tunnel: [w366] -> w311
              tunnel: [w365] -> w310
              tunnel: w305 -> [w368]
              tunnel: w297 -> [w367]
              frame #0 {
                w364 = u8 0 ("Disabled")
                n113 = property on="Transfer Start" class="Bool (strict)"("Disabled"=w364) -> ()  [unwired: 2 in, 2 out]
                n114 = VISA Write(VISA resource name=w368, write buffer=":PAGE:CHAN:MODE SWE;\n:DISP ON" ("write buffer (\"\")"), error in (no error)=w367) -> (VISA resource name out=w366:refnum<visa-resource-name>, error out=w365:errorcluster)  [unwired: 1 out]
                n115 = property on="Real time sweep" class="Bool (strict)"("Disabled"=w364) -> ()  [unwired: 2 in, 2 out]
                n116 = property on="Output Start" class="Bool (strict)"("Disabled"=w364) -> ()  [unwired: 2 in, 2 out]
                n117 = property on="QSCV Start" class="Bool (strict)"("Disabled"=w364) -> ()  [unwired: 2 in, 2 out]
              }
            }
          }
          frame 5 {
            w391 = dbl[][] []  # Array Constant
            n118 = Unbundle By Name(w405) -> ("hold time (sec)"=w402:dbl, "delay time (sec)"=w403:dbl, "Step Time (0 disables)"=w404:dbl)
            n119 = call "4155C Get Filename.vi"("error in (no error)"=w397) -> ("error out"=w395:errorcluster, "cancelled"=w394:bool, "path"=w393:path)  [unwired: 2 in]
            n120 = Bundle By Name(cluster="Drain 3", "Drain voltage"="Drain Voltage", "Drain Compliance"=w421, "Range mode"=w414, "Range"=w413) -> (w419:T3)
            n121 = control-ref of="Interrupt run"() -> (w400:refnum<vi>)
            n122 = Bundle By Name(cluster="Panel Controls 2", "Emergency Stop"=w400, "CapGraph Max"=0.001, "Text/Graph (text=false)"=TRUE) -> (w378:T1)
            n123 = Bundle By Name(cluster="Gate 3", "Gate Start"="Gate: Start 2", "Gate Stop"="Gate: Stop 2", "Gate Step"="Gate: Step 2", "Gate Compliance"=w417, "Range mode"=w416, "Range"=w415) -> (w420:T2)
            n124 = Bundle By Name(cluster="Timings 2", "hold time (sec)"=w402, "delay time (sec)"=w403, "Step Time (0 disables)"=w404, "C-Step"="Cap voltage", "CInt"="Cap I-time", "IInt"="Leak I-time") -> (w418:T4)
            n125 = stacked-sequence {
              tunnel: w378 -> [w432]
              tunnel: [w432] -> w379
              frame #0 {
                w431 = u8 2 ("Disabled")
                n126 = property on="Transfer Start" class="Bool (strict)"("Disabled"=w431) -> ()  [unwired: 2 in, 2 out]
                n127 = property on="XY Graph" class="XYGraph (strict)"("X Scale.Name Label.Text"="Vg", "Y Scale.Mapping Mode"=u8 0, "Y Scale.Name Label.Text"="Capacitance /F") -> ()  [unwired: 2 in, 2 out]
                n128 = property on="Real time sweep" class="Bool (strict)"("Disabled"=w431) -> ()  [unwired: 2 in, 2 out]
                n129 = property on="Output Start" class="Bool (strict)"("Disabled"=w431) -> ()  [unwired: 2 in, 2 out]
                n130 = property on="QSCV Start" class="Bool (strict)"("Disabled"=w431) -> ()  [unwired: 2 in, 2 out]
              }
            }
            n131 = call "4155C QSCV v3.0.vi"("VISA resource name in"=w396, "Timings"=w418, "Drain"=w419, "Gate"=w420, "Panel Controls"=w379, "error in (no error)"=w395, "QSCV - Source/Common"=w373, "QSCV - Gate"=w374, "QSCV - Drain"=w372, "QSCV - Probe 4"=w375) -> ("VISA Resource Name out"=w401:refnum<visa-resource-name>, "VG"=w383:dbl[], "Cap"=w382:dbl[], "Leak"=w385:dbl[], "error out"=w392:errorcluster)  [unwired: 4 in, 1 out]
            n132 = Bundle("VG"=w383, "Cap"=w382) -> (w381:cluster{"VG":dbl[], "Cap":dbl[]})  [unwired: 1 in]
            n133 = Build Array(w381) -> (w380:cluster{"VG":dbl[], "Cap":dbl[]}[])
            n134 = local write "XY Graph"(w380) -> ()
            n135 = Insert Into Array(array=w391, index (col)=0 ("Disabled Index (col)"), new element=w383) -> (w389:dbl[][])  [unwired: 1 in]
            n136 = Insert Into Array(array=w389, index (col)=1 ("Disabled Index (col)"), new element=w382) -> (w388:dbl[][])  [unwired: 1 in]
            n137 = Insert Into Array(array=w388, index (col)=2 ("Disabled Index (col)"), new element=w385) -> (w384:dbl[][])  [unwired: 1 in]
            n138 = case shown="False" w394 {
              tunnel: w392 -> [w442 w444]
              tunnel: [w437 w444] -> w377
              tunnel: w393 -> [w441 _]
              tunnel: w384 -> [w435 _]
              frame False {
                n139 = call <vilib>:"compatOverwrite.vi"("overwrite (F)"=TRUE) -> ("overwrite?"=w433:T14)
                n140 = Open/Create/Replace File(file path (use dialog)=w441, error in=w442, operation (0:open)=w433) -> (refnum out=w439:refnum<file>, error out=w440:errorcluster)  [unwired: 3 in, 1 out]
                n141 = call "4155C Write array to file.vi"("Byte Stream File Refnum"=w439, "Header"=string[] ["Vg /V", "Capacitance /F", "Leakage current /A"], "Data Array"=w435, "error in (no error)"=w440) -> ("dup refnum"=w436:refnum<file>, "error out"=w438:errorcluster)  [unwired: 1 in]
                n142 = Close File(refnum=w436, error in=w438) -> (error out=w437:errorcluster)  [unwired: 1 out]
              }
              frame True {
              }
            }
            n143 = stacked-sequence {
              tunnel: w377 -> [w427]
              tunnel: [w427] -> w376
              frame #0 {
                w426 = u8 0 ("Disabled")
                n144 = property on="Transfer Start" class="Bool (strict)"("Disabled"=w426) -> ()  [unwired: 2 in, 2 out]
                n145 = property on="Real time sweep" class="Bool (strict)"("Disabled"=w426) -> ()  [unwired: 2 in, 2 out]
                n146 = property on="Output Start" class="Bool (strict)"("Disabled"=w426) -> ()  [unwired: 2 in, 2 out]
                n147 = property on="QSCV Start" class="Bool (strict)"("Disabled"=w426) -> ()  [unwired: 2 in, 2 out]
              }
            }
          }
        }
      }
      n148 = call "4155C Shutdown.vi"("VISA resource name in"=w5, "error in (no error)"=w6) -> ("error out"=w8:errorcluster)  [unwired: 4 in]
      n149 = stacked-sequence {
        tunnel: w8 -> [w446]
        tunnel: [w446] -> w7
        frame #0 {
          n150 = property on="Running" class="Bool (strict)"("Boolean Text.Text"="Stopped") -> ()  [unwired: 2 in, 2 out]
        }
      }
      "error out" <- w7
    }
  }
